vi "CLSUIP_OK to Script Prop Accessors.vi"(8 "error in":errorcluster, 10 "Selected Tags":string[](array[string]), 11 "Scripters":refnum<class "BaseAccessorScripter.lvclass">[](array[class])) -> (0 "error out":errorcluster, 3 "OK to script prop accessors":bool)   [LabVIEW 2021, in "MemberVICreation.lvlib"]
uses:
  <resource>/Framework/Providers/LVClassLibrary/NewAccessors/MemberVICreation.lvlib
  <resource>/Framework/Providers/LVClassLibrary/NewAccessors/BaseAccessorScripter/BaseAccessorScripter.lvclass
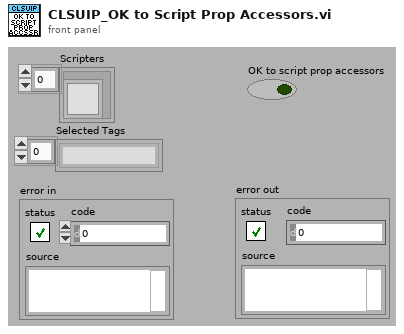
[diagram p1: front panel]
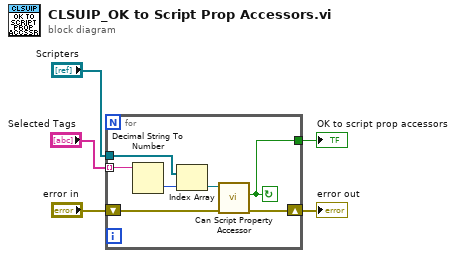
[diagram p0: block diagram]
diagram:
  n1 = for {
    tunnel: "Scripters" -> [w12]
    tunnel: [w7] -> w1
    tunnel: "Selected Tags" -> [w8] mode=indexing
    shift-right: [w9] -> w3
    shift-left: "error in" -> [w6]
    stop <- w7 continue-if-true
    n2 = Decimal String To Number(string=w8) -> (number=w11:i32)  [unwired: 2 in, 1 out]
    n3 = Index Array(array=w12, index=w11) -> (element=w10:refnum<class "BaseAccessorScripter.lvclass">)
    n4 = call-dynamic "Can Script Property Accessor.vi"("error in (no error)"=w6, "BaseAccessorScripter in"=w10) -> ("error out"=w9:errorcluster, "Can Script Property Accessor"=w7:bool)  [unwired: 7 in, 1 out]
  }
  "OK to script prop accessors" <- w1
  "error out" <- w3
